vi "Part 1.vi"(11 "Input":string) -> (3 "Output":i64)   [LabVIEW 2021]
uses:
  <userlib>/_OpenG.lib/string/string.llb/Convert EOLs (String)__ogtk.vi
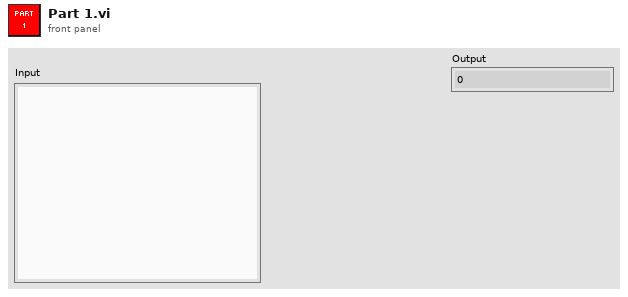
[diagram p1: front panel]
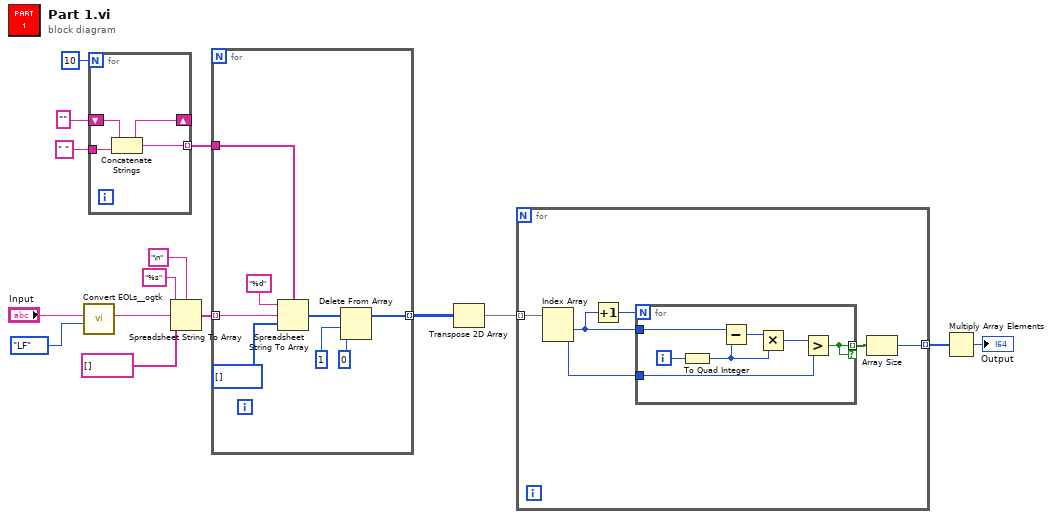
[diagram p0: block diagram]
diagram:
  n1 = call-poly <userlib>:"Convert EOLs__ogtk.vi"("Convert to:"=enum16{"CR", "LF", "CRLF"}."LF", "String in"="Input") -> ("String out"=w11:string)  [unwired: 9 in]
  n2 = for {
    N: 10 -> [_]
    tunnel: " " ("delimiter (Tab)") -> [w18]
    shift-right: [w16] -> _
    shift-left: "" -> [w17]
    tunnel: [w16] -> w5 mode=indexing
    n3 = Concatenate Strings(w17, w18) -> (w16:string)
  }
  n4 = Spreadsheet String To Array(delimiter (Tab)="\n", format string="%s", spreadsheet string=w11, array type (2D Dbl)=string[] []) -> (array=w9:string[])
  n5 = for {
    tunnel: w9 -> [w25] mode=indexing
    tunnel: w5 -> [w26]
    tunnel: [w21] -> w3 mode=indexing
    n6 = Spreadsheet String To Array(delimiter (Tab)=w26, format string="%d", spreadsheet string=w25, array type (2D Dbl)=i64[] []) -> (array=w22:i64[])
    n7 = Delete From Array(array=w22, length=1 ("index"), index=0) -> (array with subset deleted=w21:i64[])  [unwired: 1 out]
  }
  n8 = Transpose 2D Array(2D array=w3) -> (transposed array=w2:i64[][])
  n9 = for {
    tunnel: [w28] -> w4 mode=indexing
    tunnel: w2 -> [w27] mode=indexing
    n10 = Index Array(array=w27) -> (element #1=w30:i64, element #2=w31:i64)  [unwired: 2 in]
    n11 = Increment(x=w30) -> (x+1=w32:i64)
    n12 = for {
      N: w32 -> [_]
      tunnel: w31 -> [w35]
      tunnel: w30 -> [w39]
      tunnel: [w33] -> w29 mode=indexing if=w33
      i -> [w37]
      n13 = To Quad Integer(1:w37) -> (0:w34:i64)
      n14 = Subtract(x=w39, y=w34) -> (x-y=w38:i64)
      n15 = Multiply(x=w38, y=w34) -> (x*y=w36:i64)
      n16 = Greater?(x=w36, y=w35) -> (0:w33:bool)
    }
    n17 = Array Size(array=w29) -> (size(s)=w28:i32)
  }
  n18 = Multiply Array Elements(1:w4) -> (0:→"Output":i32)
